vi "createContextID.vi"(8 "error in (no error)":errorcluster, 10 "ContextID":T1, 11 "ContextIDFactory in":refnum<class "ContextIDFactory.lvclass">) -> (0 "error out":errorcluster, 2 "contextID":refnum<class "ContextID.lvclass">, 3 "ContextIDFactory out":refnum<class "ContextIDFactory.lvclass">)   [LabVIEW 2016, in "ContextIDFactory.lvclass"]
uses:
  ContextIDFactory.lvclass
  Typedefs/ContextID.ctl
  ComponentTemplateCore/ComponentModel/ComponentModel/ContextID/ContextID.lvclass
  ContextIDs/ExampleA.lvclass
  home/harini/tcs/ts_sedspectrometer/ComponentTemplateCore/ComponentModel/ComponentModel/ContextID/ContextID.lvclass
  Typedefs/SEDSpectrometerTypedefs.lvlib
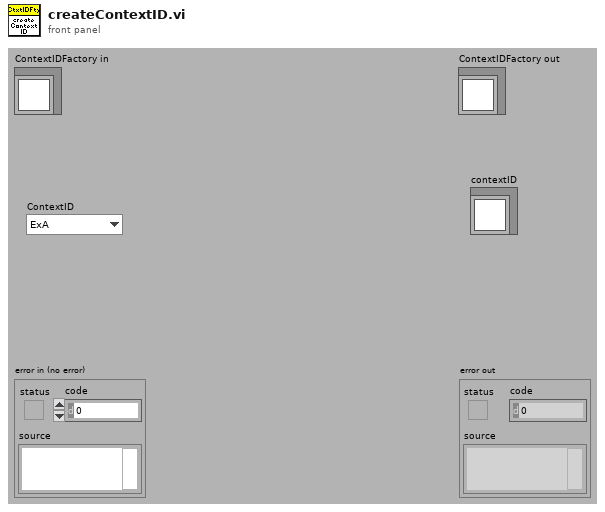
[diagram p1: front panel]
types:
  T1 = typedef "SEDSpectrometerTypedefs.lvlib/ContextID.ctl" = enum16{"ExA"}
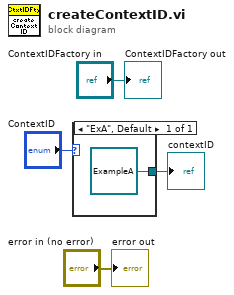
[diagram p0: block diagram]
diagram:
  n1 = case shown="\"ExA\", Default" "ContextID" {
    tunnel: [refnum<class "ExampleA.lvclass"> refnum ("A.lvclass")] -> w2
    frame "ExA", Default {
    }
  }
  "contextID" <- w2
  "error out" <- "error in (no error)"
  "ContextIDFactory out" <- "ContextIDFactory in"
